vi "FTW-Example-Actors.vi"() -> ()   [LabVIEW 2013]
uses:
  Actor/src/Connector/FTW-ActorConnector.lvclass
  Actor/src/Ether/FTW-Ether.lvclass
panel:
  out "Instance Inbox Address":string
  out "Initialized Response":string
  out "Timed out?":bool
  out "Ping Response":string
  in  "FTW Ether Configuration":string="{\n  \"ApplicationName\": \"Actor Example\",\n  \"ApplicationVersion\": \"0.1.0-1\",\n  \"LoggerAddress\": \"tcp://127.0.0.1:*\",\n  \"LoggerName\": \"ActorExample\",\n  \"LoggerDirectory\": \"[UserDesktop]\\\\Logs\",\n  \"LoggerDiskThrashDelay\": 200\n}"
  in  "Actor 1 Configuration":string="{\n  \"Identity\": \"FeatherweightActorExample\",\n  \"InboxAddress\": \"tcp://127.0.0.1:*\",\n  \"PublisherAddress\": \"tcp://127.0.0.1:*\",\n  \"DebugEnableInboxLogging\": false,\n  \"DebugEnableJobLogging\": false,\n  \"DebugShowPanel\": false\n}"
  out "error out":errorcluster
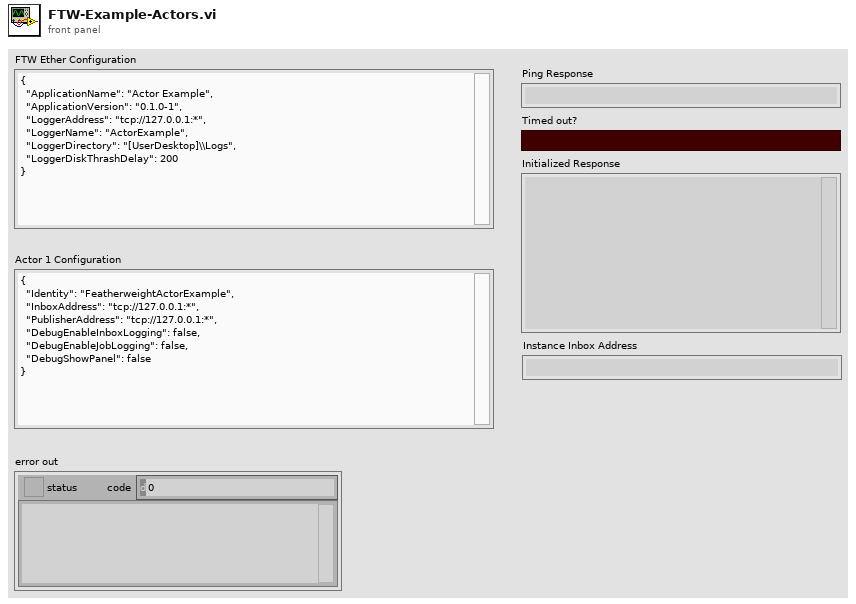
[diagram p1: front panel]
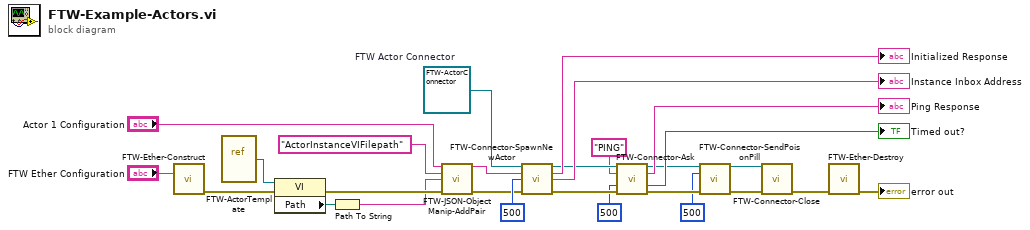
[diagram p0: block diagram]
diagram:
  w19 = refnum<class "FTW-ActorConnector.lvclass"> refnum  # FTW Actor Connector
  n1 = call "FTW-Ether-Construct.vi"("FTW Ether Configuration"="FTW Ether Configuration") -> ("error out"=w27:errorcluster)  [unwired: 14 in]
  n2 = vi-ref "FTW-ActorTemplate.vi"() -> (w18:refnum<vi>)
  n3 = property class="VI"(reference=w18, error in=w27) -> (error out=w5:errorcluster, "Path"=w2:path)  [unwired: 1 out]
  n4 = Path To String(path=w2) -> (string=w1:string)
  n5 = call "FTW-JSON-ObjectManip-AddPair.vi"("Input JSON Object"="Actor 1 Configuration", "Key"="ActorInstanceVIFilepath", "Value"=w1, "error in"=w5) -> ("Output JSON Object"=w6:string, "error out"=w4:errorcluster)  [unwired: 10 in]
  n6 = call "FTW-Connector-SpawnNewActor.vi"("FTW Actor Connector Type"=w19, "Instance Configuration"=w6, "Timeout"=500, "error in"=w4) -> ("FTW Actor Connector"=w17:refnum<class "FTW-ActorConnector.lvclass">, "Initialized Response"=→"Initialized Response":string, "Instance Inbox Address"=→"Instance Inbox Address":string, "error out"=w16:errorcluster)  [unwired: 7 in, 1 out]
  n7 = call "FTW-Connector-Ask.vi"("FTW Actor Connector"=w17, "Request Header"="PING", "Timeout"=500, "error in"=w16) -> ("FTW Actor Connector out"=w14:refnum<class "FTW-ActorConnector.lvclass">, "Response Header"=→"Ping Response":string, "Timed out?"=→"Timed out?":bool, "error out"=w13:errorcluster)  [unwired: 7 in, 1 out]
  n8 = call-dynamic "FTW-Connector-SendPoisonPill.vi"("FTW Actor Connector"=w14, "Timeout"=500, "error in"=w13) -> ("FTW Actor Connector out"=w12:refnum<class "FTW-ActorConnector.lvclass">, "error out"=w11:errorcluster)  [unwired: 8 in, 3 out]
  n9 = call-dynamic "FTW-Connector-Close.vi"("FTW Actor Connector"=w12, "error in"=w11) -> ("error out"=w23:errorcluster)  [unwired: 13 in]
  n10 = call "FTW-Ether-Destroy.vi"("error in"=w23) -> ("error out"=→"error out":errorcluster)  [unwired: 14 in]
